vi "UtilsStr_ParseStringToArray.vi"(2 "DeleteConsecutiveDelimiter":bool, 3 "Delimiter":string, 4 "InputString":string) -> (1 "Array":string[](array[string]))   [LabVIEW 2013]
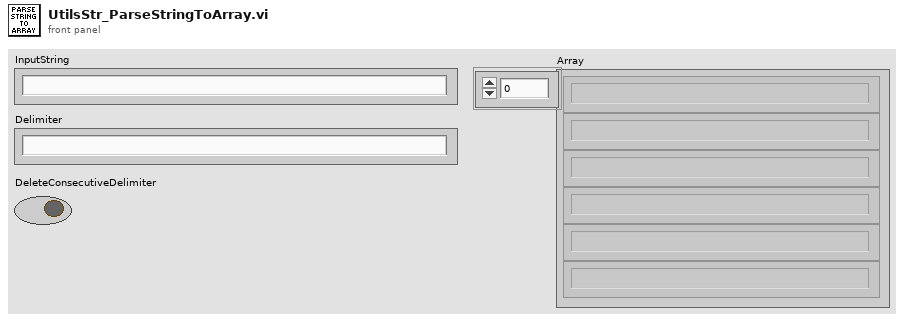
[diagram p1: front panel]
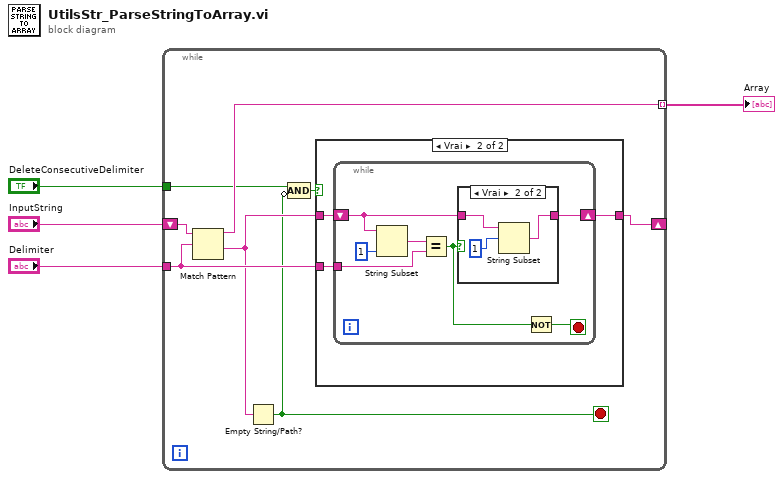
[diagram p0: block diagram]
diagram:
  n1 = while {
    shift-right: [w8] -> _
    shift-left: "InputString" -> [w12]
    tunnel: "Delimiter" -> [w10]
    tunnel: [w11] -> w2 mode=indexing
    tunnel: "DeleteConsecutiveDelimiter" -> [w7]
    stop <- w6 stop-if-true
    n2 = Match Pattern(string=w12, regular expression=w10) -> (before substring=w11:string, after substring=w9:string)  [unwired: 1 in, 2 out]
    n3 = Empty String/Path?(string/path=w9) -> (empty?=w6:bool)
    n4 = Compound Arithmetic op=AND(w7, invert w6) -> (w5:bool)
    n5 = case shown="Vrai" w5 {
      tunnel: w9 -> [w13 w16]
      tunnel: w10 -> [_ w15]
      tunnel: [w13 w14] -> w8
      frame False {
      }
      frame True {
        n6 = while {
          shift-right: [w20] -> w14
          shift-left: w16 -> [w17]
          tunnel: w15 -> [w21]
          stop <- w19 stop-if-true
          n7 = String Subset(string=w17, length (rest)=1 ("longueur (reste)")) -> (substring=w22:string)  [unwired: 1 in]
          n8 = Equal?(x=w22, y=w21) -> (x = y?=w18:bool)
          n9 = case shown="Vrai" w18 {
            tunnel: [w24 w26] -> w20
            tunnel: w17 -> [w24 w25]
            frame False {
            }
            frame True {
              n10 = String Subset(string=w25, offset (0)=1 ("longueur (reste)")) -> (substring=w26:string)  [unwired: 1 in]
            }
          }
          n11 = Not(x=w18) -> (.not. x?=w19:bool)
        }
      }
    }
  }
  "Array" <- w2
